vi "HandleRollerMotor.vi"(5 "OffState":T1, 7 "ReverseState":T1, 8 "error in":errorcluster, 9 "JoystickValue":dbl, 11 "ForwardState":T1) -> (0 "error out":errorcluster, 2 "StateOut":T1, 3 "Enqueue?":bool)   [LabVIEW 2013]
doc: "If Joystick Values is not equal to 0 then if it is > 0 do Forward State. if < 0 then ReverseState.\nOtherwiae go to OffState"
uses:
  RollerAction.ctl
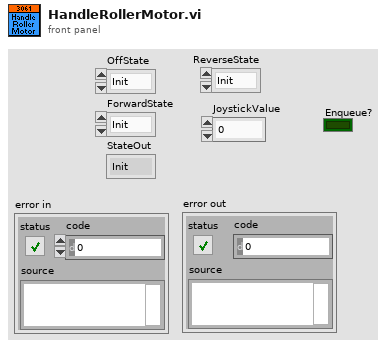
[diagram p1: front panel]
types:
  T1 = typedef "RollerAction.ctl" = enum16{"Init", "Off", "Forward", "Reverse"}
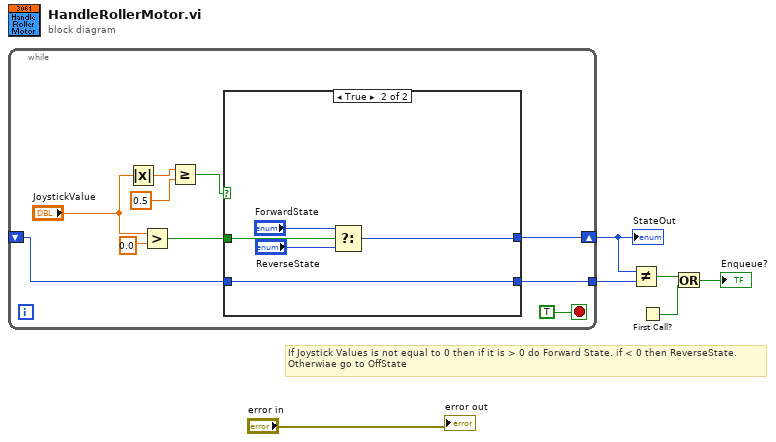
[diagram p0: block diagram]
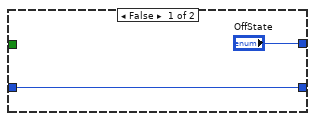
[diagram p2: hidden frame]
diagram:
  # "If Joystick Values is not equal to 0 then if it is > 0 do Forward State. if < 0 then ReverseState.\nOtherwiae go to OffState"
  n1 = while {
    shift-right: [w10] -> w5
    shift-left: _ -> [w8]
    tunnel: [w7] -> w4
    stop <- TRUE stop-if-true
    n2 = Absolute Value(x="JoystickValue") -> (abs(x)=w13:dbl)
    n3 = Greater?(x="JoystickValue", y=0.0) -> (0:w15:bool)
    n4 = Greater Or Equal?(x=w13, y=0.5) -> (x >= y?=w11:bool)
    n5 = case shown="True" w11 {
      tunnel: ["OffState" w23] -> w10
      tunnel: w15 -> [_ w22]
      tunnel: w8 -> [w17 w19]
      tunnel: [w17 w19] -> w7
      frame False {
      }
      frame True {
        n6 = Select(t="ForwardState", s=w22, f="ReverseState") -> (s? t:f=w23:T1)
      }
    }
  }
  "StateOut" <- w5
  n7 = Not Equal?(x=w5, y=w4) -> (x != y?=w3:bool)
  n8 = First Call?() -> (First Call?: T/F=w2:bool)
  n9 = Or(x=w3, y=w2) -> (x .or. y?=→"Enqueue?":bool)
  "error out" <- "error in"
